vi "VI Tree.vi"   [LabVIEW 2012, in "Phidget Voltage Output.lvlib"]
doc: "${VoltageOutput:VITreeHeader}"
uses:
  <instrlib>/Phidgets/Phidget Voltage Output/Phidget Voltage Output.lvlib
  <instrlib>/Phidgets/Phidget Voltage Output/Public/VoltageOutputStart.vi
  <instrlib>/Phidgets/Phidget Voltage Output/Public/VoltageOutputOpen.vi
  <instrlib>/Phidgets/Phidget Voltage Output/Public/VoltageOutputClose.vi
panel:
  # "(c) 2015 Phidgets Inc..  ALL RIGHTS RESERVED."
  # "SEE DIAGRAM\nFOR VI TREE."
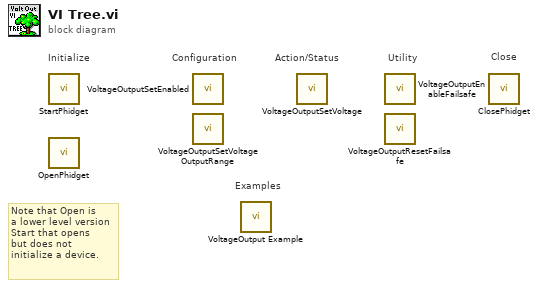
[diagram p0: block diagram]
diagram:
  # "Utility"
  # "Note that Open is\na lower level version\nStart that opens\nbut does not \ninitialize a device."
  # "Examples"
  # "Configuration"
  # "Action/Status"
  # "Close"
  # "Initialize"
  n1 = call-poly <instrlib>:"StartPhidget.vi"() -> ()  [unwired: 12 in, 4 out]
  n2 = call-poly <instrlib>:"OpenPhidget.vi"() -> ()  [unwired: 8 in, 4 out]
  n3 = call <instrlib>:"VoltageOutputSetEnabled.vi"() -> ()  [unwired: 9 in, 2 out]
  n4 = call <instrlib>:"VoltageOutputSetVoltageOutputRange.vi"() -> ()  [unwired: 9 in, 2 out]
  n5 = call <instrlib>:"VoltageOutput Example.vi"() -> ()  [unwired: 12 in]
  n6 = call <instrlib>:"VoltageOutputSetVoltage.vi"() -> ()  [unwired: 9 in, 2 out]
  n7 = call <instrlib>:"VoltageOutputEnableFailsafe.vi"() -> ()  [unwired: 9 in, 2 out]
  n8 = call <instrlib>:"VoltageOutputResetFailsafe.vi"() -> ()  [unwired: 9 in, 2 out]
  n9 = call-poly <instrlib>:"ClosePhidget.vi"() -> ()  [unwired: 11 in, 1 out]
